vi "state control.vi"(8 "Data Status":T1, 9 "Plant Method":T2={"Operator information"=[], "data log interval"=60, "data loop interval"=10, "Datalog directory path"=path "", "graph update interval"=1.0, "history length"=1000, "Control Logic file path"=path "", "Sensor Configuration file path"=path "", "HMI VI path"=path "", "HMI data smooth"=5.0} {"HMI data smooth" min=0.01 format="%.2f"; "history length" min=1; "graph update interval" min=0.1 format="%.2f"; "data log interval" min=1}, 10 "Plant Mode of Operation":T4=enum."Automatic Operation", 11 "Operator Selected State":u16(ring)=1) -> (1 "Elapsed time in current state":dbl format="%.2f", 3 "Plant State out":u16(ring)=1)   [LabVIEW 2012]
uses:
  Plant mode.ctl
  Plant method.ctl
  operator info.ctl
  data status.ctl
  DAQ configuration/Sensor buffer command.ctl
  logic buffer cmd.ctl
panel:
  in  "Tab Control":enum32{"Inputs", "Outputs"}(tab)
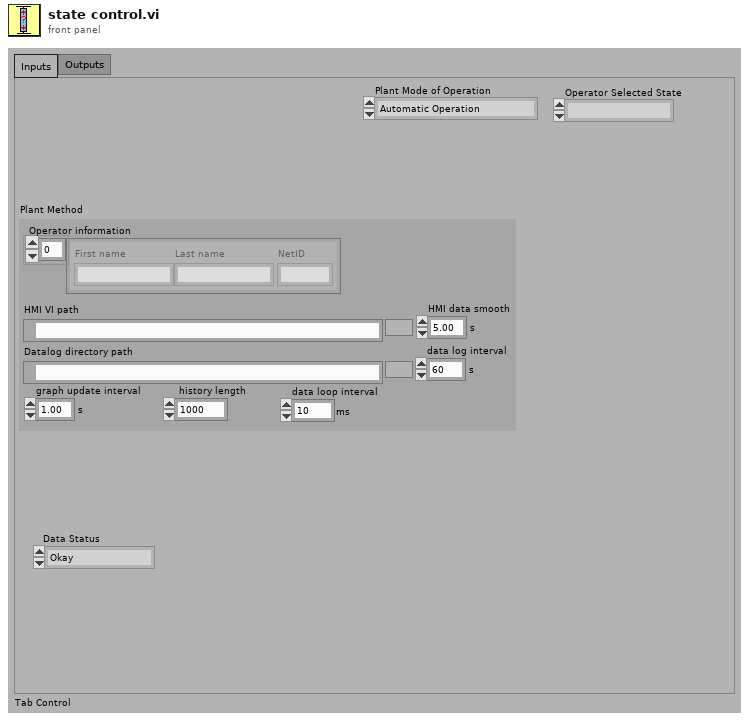
[diagram p1: front panel]
types:
  T1 = typedef "data status.ctl" = enum16{"Okay", "Sensor Range error", "Server error"}
  T2 = typedef "Plant method.ctl" = cluster{"Operator information":T3, "data log interval":u32, "data loop interval":u32, "Datalog directory path":path, "graph update interval":sgl, "history length":u16, "Control Logic file path":path, "Sensor Configuration file path":path, "HMI VI path":path, "HMI data smooth":dbl}
  T3 = typedef "operator info.ctl" = cluster{"First name":string, "Last name":string, "NetID":string}[]
  T4 = typedef "Plant mode.ctl" = enum16{"Manual Locked in State", "Automatic Operation"}
  T5 = typedef "logic buffer cmd.ctl" = enum16{"read", "write ouput settings", "write rules", "write setpoints", "write output descriptions", "write all", "calculate setpoints", "save", "open", "Load all setpoint code", "Load one setpoint code", "Configure one setpoint code"}
  T6 = typedef "Sensor buffer command.ctl" = enum16{"read average", "read recent", "read all", "write", "configure", "clear"}
  T7 = typedef "Sensor data.ctl" = cluster{" Sensor array":T8[], "Time":dbl}
  T8 = typedef "sensor cluster.ctl" = cluster{"voltage":sgl, "scaled":sgl, "units":string, "Out of Range":bool}
  T9 = typedef "Plant state.ctl" = u16
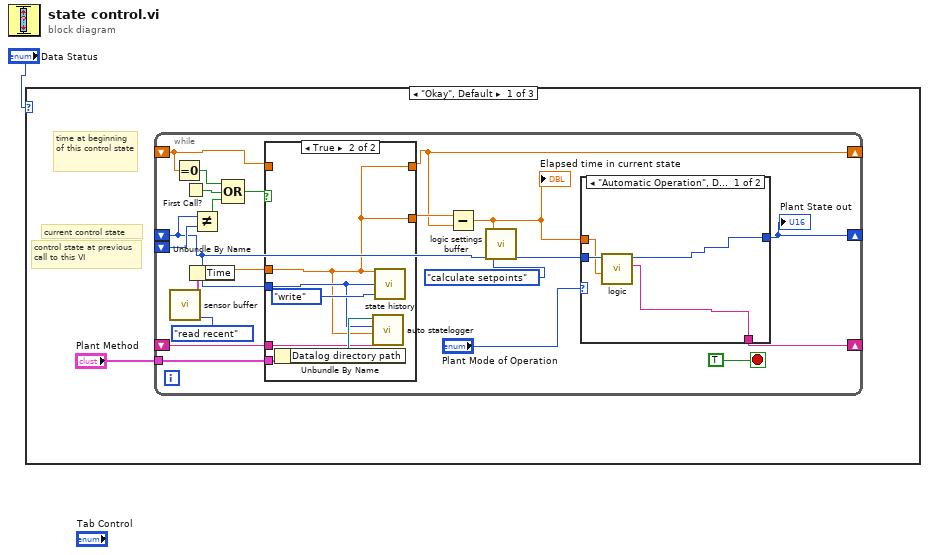
[diagram p0: block diagram]
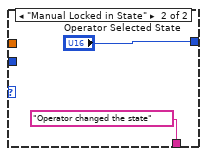
[diagram p3: hidden frame]
diagram:
  n1 = case shown="\"Okay\", Default" "Data Status" {
    frame "Okay", Default {
      # "current control state"
      # "control state at previous call to this VI"
      # "time at beginning of this control state"
      n2 = while {
        tunnel: "Plant Method" -> [w19]
        shift-left: _ -> [w13]
        shift-right: [w14] -> _
        shift-left: _ -> [w20]
        shift-left: _ -> [w4]
        shift-right: [w7] -> _
        shift-right: [w8] -> _
        shift-left: _ -> [w17]
        stop <- TRUE stop-if-true
        n3 = call "sensor buffer.vi"("command"=Sensor_buffer_command."read recent") -> ("Sensor Data smoothed"=w21:T7)  [unwired: 4 in, 2 out]
        n4 = Equal To 0?(x=w13) -> (x = 0?=w12:bool)
        n5 = First Call?() -> (First Call?: T/F=w11:bool)
        n6 = Unbundle By Name(w21) -> ("Time"=w16:dbl)
        n7 = Not Equal?(x=w4, y=w20) -> (x != y?=w10:bool)
        n8 = Compound Arithmetic op=OR(w12, w11, w10) -> (w9:bool)
        n9 = case shown="True" w9 {
          tunnel: w16 -> [w25 w26]
          tunnel: w4 -> [_ w28]
          tunnel: w19 -> [_ w30]
          tunnel: w17 -> [_ w27]
          tunnel: [w25 w26] -> w15
          tunnel: [w24 w26] -> w14
          tunnel: w13 -> [w24 _]
          frame False {
          }
          frame True {
            n10 = Unbundle By Name(w30) -> ("Datalog directory path"=w29:path)
            n11 = call "auto statelogger.vi"("Rule name"=w27, "Time"=w26, "Plant State"=w28, "Datalog directory path"=w29) -> ()  [unwired: 7 in, 1 out]
            n12 = call "state history.vi"("command"=enum16{"write", "read", "reset"}."write", "Plant State"=w28, "Time"=w26) -> ()  [unwired: 1 out]
          }
        }
        n13 = Subtract(x=w15, y=w14) -> (x-y=w5:dbl)
        "Elapsed time in current state" <- w5
        n14 = call "logic settings buffer.vi"("Plant  state"=w4, "Elapsed time in current state"=w5, "command"=logic_buffer_cmd."calculate setpoints") -> ("Plant  state out"=w3:u16)  [unwired: 9 in, 7 out]
        n15 = case shown="\"Automatic Operation\", Default" "Plant Mode of Operation" {
          tunnel: [w33 "Operator Selected State"] -> w7
          tunnel: w3 -> [w35 _]
          tunnel: w5 -> [w34 _]
          tunnel: [w32 "Operator changed the state" ("Rule name")] -> w8
          frame "Automatic Operation", Default {
            n16 = call "logic.vi"("Elapsed time in current state"=w34, "Plant State in"=w35) -> ("Rule name"=w32:string, "Plant State out"=w33:T9)  [unwired: 8 in]
          }
          frame "Manual Locked in State" {
          }
        }
        "Plant State out" <- w7
      }
    }
    frame "Sensor Range error" {
    }
    frame "Server error" {
    }
  }
